vi "Get New Position.vi"(10 "Direction":T1, 11 "Formics in":refnum<class "Formics.lvclass">) -> (2 "MyPosition":cluster{"X":i32, "Y":i32}, 3 "Formics out":refnum<class "Formics.lvclass">)   [LabVIEW 2015, in "Formics.lvclass"]
uses:
  Formics.lvclass
  Type Defs/Direction Enum.ctl
  Formics.lvclass/Formics.ctl
  Type Defs/SB Type Defs.lvlib
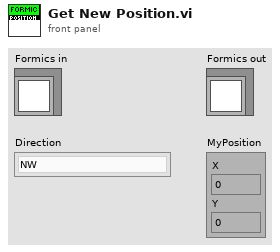
[diagram p1: front panel]
types:
  T1 = typedef "SB Type Defs.lvlib/Direction Enum.ctl" = enum16{"NW", "N", "NE", "E", "SE", "S", "SW", "W"}
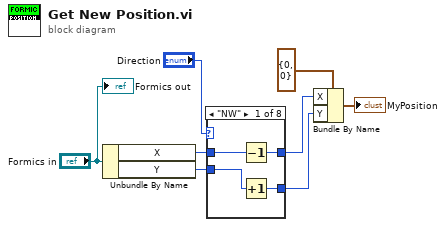
[diagram p0: block diagram]
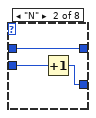
[diagram p2: hidden frame]
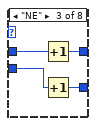
[diagram p3: hidden frame]
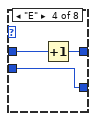
[diagram p4: hidden frame]
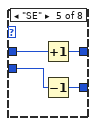
[diagram p5: hidden frame]
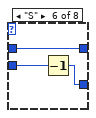
[diagram p6: hidden frame]
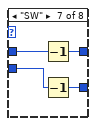
[diagram p7: hidden frame]
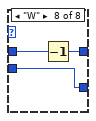
[diagram p8: hidden frame]
diagram:
  n1 = Unbundle By Name("Formics in") -> ("X"=w3:i32, "Y"=w4:i32)
  n2 = case shown="\"NW\"" "Direction" {
    tunnel: w3 -> [w12 w15 w19 w22 w26 w29 w33 w36]
    tunnel: w4 -> [w11 w14 w18 w21 w25 w28 w32 w35]
    tunnel: [w10 w15 w16 w20 w24 w29 w30 w34] -> w6
    tunnel: [w9 w13 w17 w21 w23 w27 w31 w35] -> w7
    frame "NW" {
      n3 = Decrement(x=w12) -> (x-1=w10:i32)
      n4 = Increment(x=w11) -> (x+1=w9:i32)
    }
    frame "N" {
      n5 = Increment(x=w14) -> (x+1=w13:i32)
    }
    frame "NE" {
      n6 = Increment(x=w19) -> (x+1=w16:i32)
      n7 = Increment(x=w18) -> (x+1=w17:i32)
    }
    frame "E" {
      n8 = Increment(x=w22) -> (x+1=w20:i32)
    }
    frame "SE" {
      n9 = Increment(x=w26) -> (x+1=w24:i32)
      n10 = Decrement(x=w25) -> (x-1=w23:i32)
    }
    frame "S" {
      n11 = Decrement(x=w28) -> (x-1=w27:i32)
    }
    frame "SW" {
      n12 = Decrement(x=w33) -> (x-1=w30:i32)
      n13 = Decrement(x=w32) -> (x-1=w31:i32)
    }
    frame "W" {
      n14 = Decrement(x=w36) -> (x-1=w34:i32)
    }
  }
  n15 = Bundle By Name(cluster=cluster{"X":i32, "Y":i32} {"X"=0, "Y"=0} ("MyPosition"), "X"=w6, "Y"=w7) -> (→"MyPosition":cluster{"X":i32, "Y":i32})
  "Formics out" <- "Formics in"
